vi "ReadDisplayImage.vi"(11 "Picture in":refnum<vi>) -> (3 "Overview":picture)   [LabVIEW 2024]
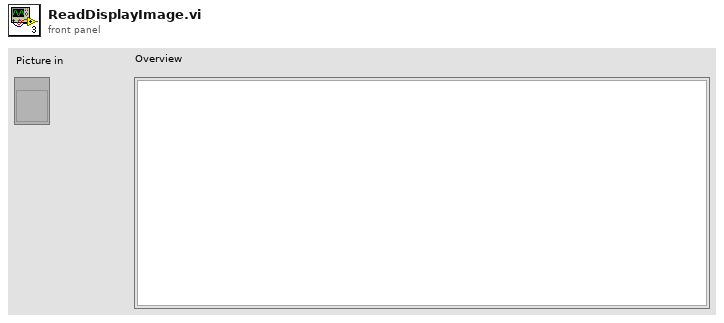
[diagram p1: front panel]
types:
  T1 = typedef "LVBoundsTypeDef.ctl" = cluster{"Width":u32, "Height":u32}
  T2 = typedef "imagedata.ctl" = cluster{"image type":i32, "image depth":i32, "image":u8[], "mask":u8[], "colors":u32[], "Rectangle":cluster{"left":i16, "top":i16, "right":i16, "bottom":i16}}
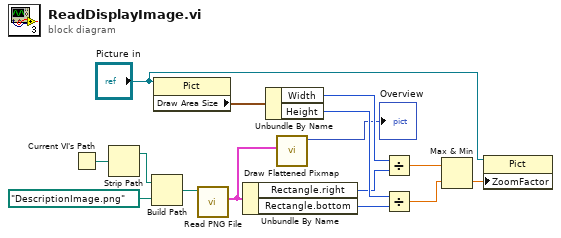
[diagram p0: block diagram]
diagram:
  n1 = Current VI's Path() -> (path=w5:path)
  n2 = Strip Path(path=w5) -> (stripped path=w6:path)  [unwired: 1 out]
  n3 = Build Path(base path=w6, name or relative path=path "DescriptionImage.png") -> (appended path=w3:path)
  n4 = property on="Property Node" class="Pict"(reference="Picture in") -> ("Draw Area Size"=w7:T1)  [unwired: 1 in, 2 out]
  n5 = call <vilib>:"Read PNG File.vi"("path to PNG file"=w3) -> ("image data"=w8:T2)  [unwired: 8 in, 2 out]
  n6 = Unbundle By Name(w8) -> ("Rectangle.right"=w10:i16, "Rectangle.bottom"=w11:i16)
  n7 = Unbundle By Name(w7) -> ("Width"=w9:u32, "Height"=w12:u32)
  n8 = call <vilib>:"Draw Flattened Pixmap.vi"("image data"=w8) -> ("new picture"=→"Overview":picture)  [unwired: 8 in]
  n9 = Divide(x=w9, y=w10) -> (x/y=w13:dbl)
  n10 = Divide(x=w12, y=w11) -> (x/y=w14:dbl)
  n11 = Max & Min(x=w13, y=w14) -> (min(x,y)=w15:dbl)  [unwired: 1 out]
  n12 = property on="Property Node" class="Pict"(reference="Picture in", "ZoomFactor"=w15) -> ()  [unwired: 1 in, 2 out]
